vi "SetLoggerLevel.vi"(8 "error in (no error)":errorcluster, 10 "Level":T1=enum."WARNING", 11 "Logger in":refnum<class "Logger.lvclass">) -> (0 "error out":errorcluster, 3 "Logger out":refnum<class "Logger.lvclass">)   [LabVIEW 2022 SP3, in "Logger.lvlib" / "Logger.lvclass"]
uses:
  Logger.lvclass
  C:/Users/jakub/repos/gh/sw4sys/lv-logger/PythonWrapper/Source/PythonWrapper/PythonWrapper.lvclass
  C:/Users/jakub/repos/gh/sw4sys/lv-logger/Logger/Source/LoggingWrapper/LoggingWrapper.lvclass
  _Level.ctl
  PythonWrapper/Source/PythonWrapper/PythonWrapper.lvclass/PythonWrapper.ctl
  LoggingWrapper/LoggingWrapper.lvclass/LoggingWrapper.ctl
  Logger.lvclass/Logger.ctl
  PythonWrapper/Source/PythonWrapper/Read PythonSession.vi
  PythonWrapper/Source/PythonWrapper/Read ModulePath.vi
  Read Name.vi
  Write Level.vi
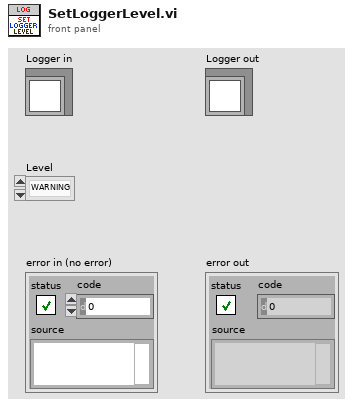
[diagram p1: front panel]
types:
  T1 = typedef "Logger.lvlib/Logger.lvclass/_Level.ctl" = enum16{"NOTSET", "DEBUG", "INFO", "WARNING", "ERROR", "CRITICAL"}
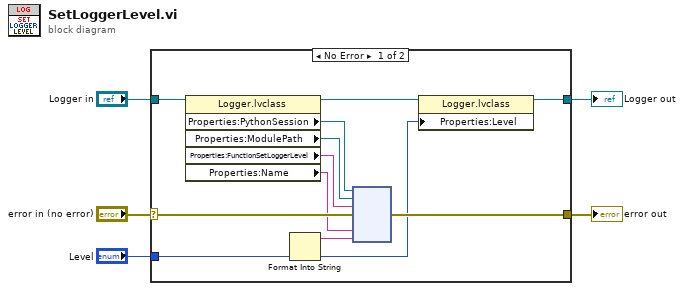
[diagram p0: block diagram]
diagram:
  n1 = case shown="No Error" "error in (no error)" {
    selector: "error in (no error)" -> [w14 w18]
    tunnel: [w13 w18] -> w4
    tunnel: [w9 w17] -> w2
    tunnel: "Logger in" -> [w16 w17]
    tunnel: "Level" -> [w8 _]
    frame No Error {
      n2 = property class="Logger.lvclass"(reference=w16) -> (reference out=w15:refnum<class "Logger.lvclass">, "Properties:PythonSession"=w12:refnum<k35>, "Properties:ModulePath"=w10:path, "Properties:FunctionSetLoggerLevel"=w11:string, "Properties:Name"=w6:string)  [unwired: 1 in, 1 out]
      n3 = Format Into String(w8) -> (resulting string=w7:string)  [unwired: 3 in, 1 out]
      n4 = node(w12, w10, w11, w14, w6, w7) -> (w13:errorcluster)  [unwired: 4 in, 3 out]
      n5 = property class="Logger.lvclass"(reference=w15, "Properties:Level"=w8) -> (reference out=w9:refnum<class "Logger.lvclass">)  [unwired: 1 in, 1 out]
    }
    frame Error {
    }
  }
  "error out" <- w4
  "Logger out" <- w2
